vi "sonde data write to excel.vi"() -> ()   [LabVIEW 2016]
uses:
  Groundwater header.ctl
  activeXtest/activeXtest 2015 Folder/sample data row cluster.ctl
  activeXtest/activeXtest 2015 Folder/sonde cluster.ctl
  <vilib>/Utility/NIReport.llb/NI_report.lvclass
panel:
  out "Current Sample Sheet":string
  in  "stop":bool
  out "row max value":i32
  in  "Write Data Line":bool
  out "last occupied cell's name":string
  in  "Final Data for Sample Sheet?":bool
  in  "Sample Sheet Data Row Cluster":T1={"Head"=0.0, "Depth"=0.0, "comment string"="", "Sonde Data Cluster"={"Cumulative\nVolume"=100.0, "Specific\nConductance"=2.0, "Dissolved\nOxygen"=3.0, "pH"=4.0, "ORP"=5.0, "Temp"=26.0, "Salinity"=7.0}} {"Sonde Data Cluster"."Salinity" format="%_3g"; "Sonde Data Cluster"."Temp" format="%_2g"; "Sonde Data Cluster"."ORP" format="%_4g"; "Sonde Data Cluster"."pH" format="%_4g"; "Sonde Data Cluster"."Dissolved\nOxygen" format="%_4g"; "Sonde Data Cluster"."Specific\nConductance" format="%_4g"; "Sonde Data Cluster"."Cumulative\nVolume" format="%#_4g"}
  out "number of rows":i32
  in  "report file path 2":path=path "D:/Cascade/templates/Groundwater Profiling Log_empty_2.xlsx"
  out "data":string[][](array[string])
  out "Elapsed Time (ms)":u32
  in  "error in (no error)":errorcluster
  in  "Groundwater Header":T3
  out "Worksheet Names":string[](array[string])
  in  "template file path":path=path "D:/Cascade/templates/Groundwater Profiling Log_empty_labview_template.xlsx"
  out "error out":errorcluster
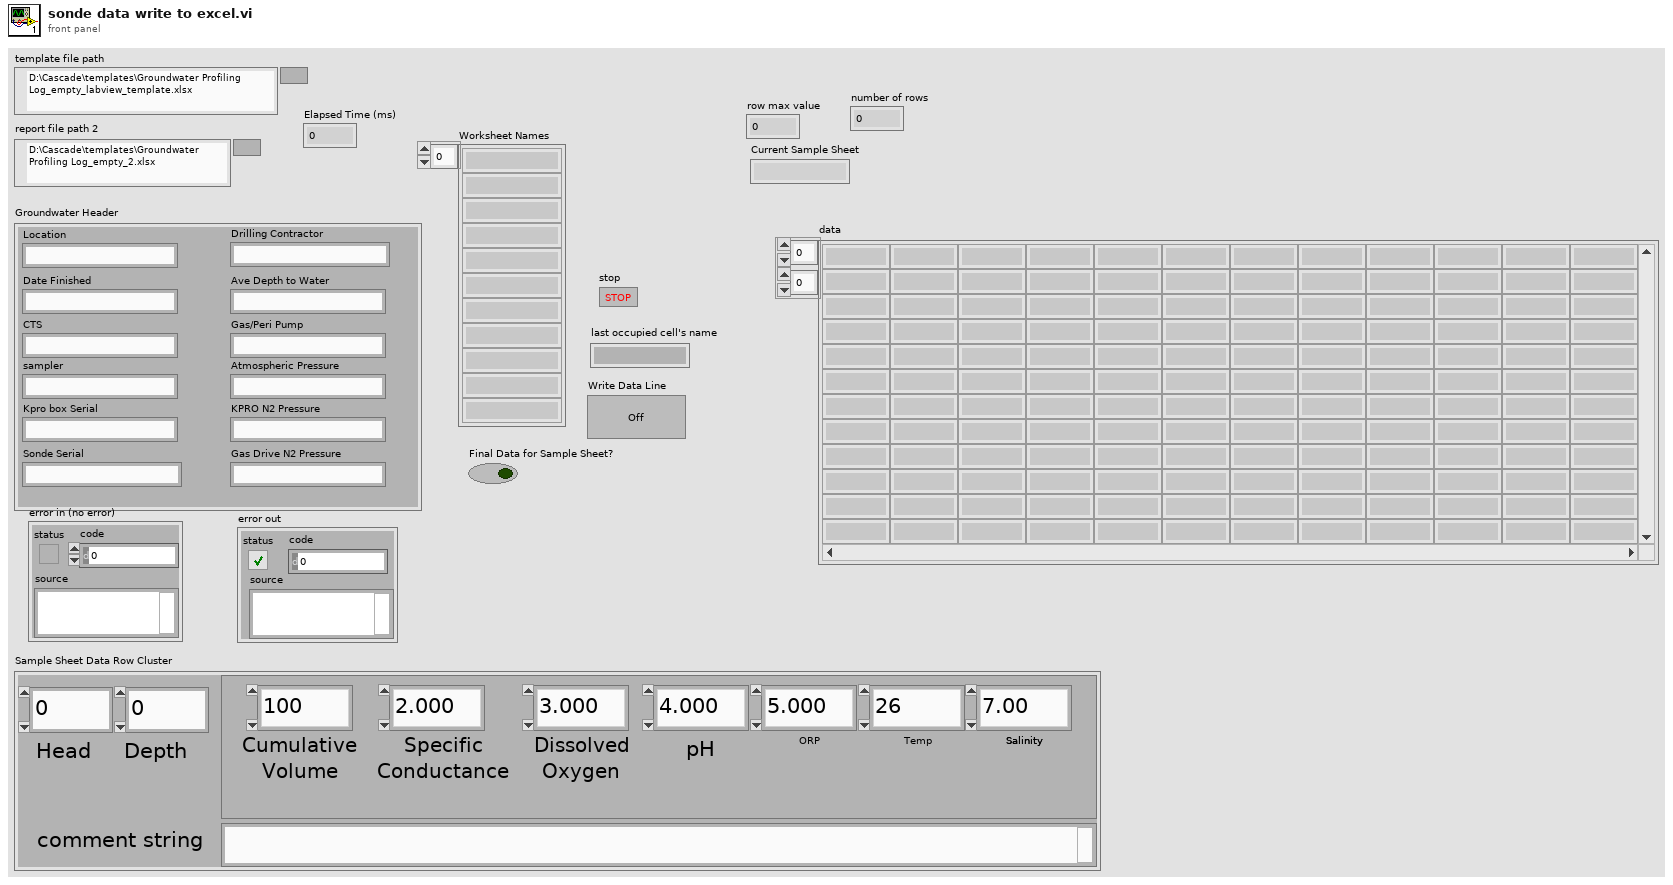
[diagram p1: front panel]
types:
  T1 = typedef "sample data row cluster.ctl" = cluster{"Head":dbl, "Depth":dbl, "comment string":string, "Sonde Data Cluster":T2}
  T2 = typedef "sonde cluster.ctl" = cluster{"Cumulative\nVolume":dbl, "Specific\nConductance":dbl, "Dissolved\nOxygen":dbl, "pH":dbl, "ORP":dbl, "Temp":dbl, "Salinity":dbl}
  T3 = typedef "Groundwater header.ctl" = cluster{"Location":string, "Date Finished":string, "CTS":string, "sampler":string, "Kpro box Serial ":string, "Sonde Serial":string, "Drilling Contractor":string, "Ave Depth to Water":string, "Gas/Peri Pump":string, "Atmospheric Pressure":string, "KPRO N2 Pressure":string, "Gas Drive N2 Pressure":string}
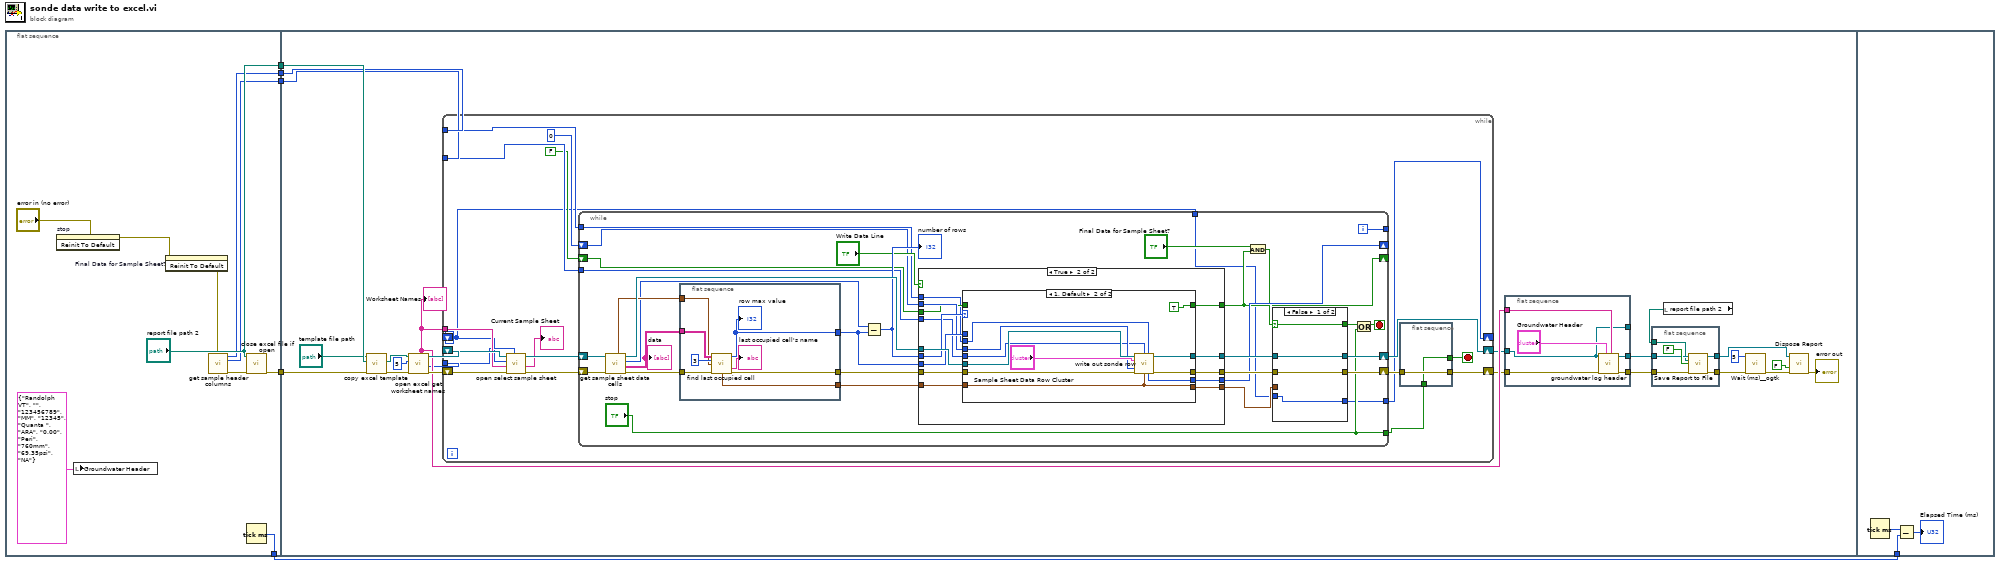
[diagram p0: block diagram]
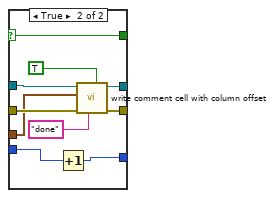
[diagram p4: hidden frame]
diagram:
  n1 = flat-sequence {
    tunnel: [w14] -> w5
    tunnel: [w12] -> w4
    tunnel: ["report file path 2"] -> w3
    tunnel: [w10] -> w2
    tunnel: [w9] -> w1
    tunnel: w4 -> [w26]
    tunnel: w3 -> [w24]
    tunnel: w2 -> [w19]
    tunnel: w1 -> [w18]
    tunnel: w5 -> [w161]
    frame #0 {
      n2 = invoke on="stop" class="Bool" method="Reinit To Default"(error in="error in (no error)") -> (error out=w6:errorcluster)  [unwired: 2 in, 2 out]
      n3 = local write "Groundwater Header"(T3 {"Location"="Randolph VT", "Date Finished"="", "CTS"="123456789", "sampler"="MM", "Kpro box Serial "="12345", "Sonde Serial"="Quanta ", "Drilling Contractor"="ARA", "Ave Depth to Water"="0.00", "Gas/Peri Pump"="Peri", "Atmospheric Pressure"="760mm", "KPRO N2 Pressure"="69.35psi", "Gas Drive N2 Pressure"="NA"} ("Groundwater Header 2")) -> ()
      n4 = invoke on="Final Data for Sample Sheet?" class="Bool" method="Reinit To Default"(error in=w6) -> (error out=w11:errorcluster)  [unwired: 2 in, 2 out]
      n5 = call "get sample header columns.vi"("error in (no error)"=w11) -> ("Column of Volume"=w10:i32, "Columns"=w9:i32[], "error out"=w8:errorcluster)  [unwired: 5 in, 7 out]
      n6 = call "close excel file if open.vi"("error in (no error)"=w8, "report file path in"="report file path 2") -> ("error out"=w12:errorcluster)  [unwired: 8 in, 1 out]
      n7 = Tick Count (ms)() -> (millisecond timer value=w14:u32)
    }
    frame #1 {
      n8 = call "copy excel template.vi"("error in (no error)"=w26, "report file path in"=w24, "template file path in"="template file path") -> ("error out"=w22:errorcluster, "report file path out"=w25:path)  [unwired: 7 in]
      n9 = call "open excel get worksheet names.vi"("error in (no error)"=w22, "milliseconds to wait"=u32 5, "report file path"=w25) -> ("error out"=w32:errorcluster, "Number of Sample Sheets"=w17:i32, "NI_report out"=w31:refnum<class "NI_report.lvclass">, "Worksheet Names"=w29:string[])  [unwired: 3 in, 2 out]
      "Worksheet Names" <- w29
      n10 = while {
        tunnel: w29 -> [w54]
        tunnel: w19 -> [w51]
        tunnel: w18 -> [w50]
        tunnel: w17 -> [w49]
        shift-right: [w45] -> w21
        shift-left: w32 -> [w56]
        shift-right: [w52] -> w20
        shift-left: w31 -> [w55]
        shift-right: [w41] -> _
        shift-left: 1 ("input 1") -> [w40]
        stop <- w48 stop-if-true
        n11 = call "open select sample sheet.vi"("Number of Sample Sheets"=w49, "error in (no error)"=w56, "Worksheet Names"=w54, "Active Sample Sheet"=w40, "NI_report in"=w55) -> ("error out"=w53:errorcluster, "Current Sample Sheet"=→"Current Sample Sheet":string, "NI_report out"=w57:refnum<class "NI_report.lvclass">)  [unwired: 4 in]
        n12 = while {
          shift-right: [w75] -> w52
          shift-left: w57 -> [w88]
          shift-right: [w77] -> w46
          shift-left: w53 -> [w79]
          tunnel: [w72] -> _
          shift-right: [w70] -> _
          shift-left: 0 ("row index") -> [w71]
          shift-right: [w64] -> _
          shift-left: FALSE ("x") -> [w67]
          tunnel: w51 -> [w66]
          tunnel: w50 -> [w65]
          tunnel: ["stop"] -> w44
          tunnel: w40 -> [w59]
          tunnel: [w58] -> w41
          i -> [w72]
          stop <- w61 stop-if-true
          n13 = call "get sample sheet data cells.vi"("error in (no error)"=w79, "NI_report in"=w88) -> ("error out"=w86:errorcluster, "data"=w80:string[][], "row"=w84:i32, "NI_report out"=w87:refnum<class "NI_report.lvclass">, "output cluster"=w85:cluster{"row":i32, "column":i32})  [unwired: 5 in]
          "data" <- w80
          n14 = flat-sequence {
            tunnel: w86 -> [w145]
            tunnel: w80 -> [w144]
            tunnel: w85 -> [w142]
            tunnel: [w141] -> w82
            tunnel: [w140] -> w81
            tunnel: [w139] -> w74
            frame #0 {
              n15 = call "find last occupied cell.vi"("data"=w144, "Header Rows to remove"=3, "sub array start"=w142, "error in (no error)"=w145) -> ("row max value"=w140:i32, "last occupied cell's name"=→"last occupied cell's name":string, "start of last occupied row"=w139:cluster{"row":i32, "column":i32}, "error out"=w141:errorcluster)  [unwired: 5 in, 3 out]
              "row max value" <- w140
            }
          }
          n16 = Subtract(x=w84, y=w81) -> (x-y=w83:i32)
          "number of rows" <- w83
          n17 = case shown="True" "Write Data Line" {
            tunnel: w87 -> [w93 w107]
            tunnel: w83 -> [_ w106]
            tunnel: w82 -> [w92 w105]
            tunnel: w81 -> [_ w104]
            tunnel: [w92 w103] -> w78
            tunnel: [w93 w102] -> w76
            tunnel: w74 -> [w90 w101]
            tunnel: w71 -> [w91 w100]
            tunnel: [w91 w99] -> w70
            tunnel: [w90 w98] -> w68
            tunnel: w67 -> [w89 w97]
            tunnel: [w89 w96] -> w64
            tunnel: w66 -> [_ w95]
            tunnel: w65 -> [_ w94]
            frame False {
            }
            frame True {
              n18 = case shown="1, Default" w106 {
                tunnel: [w111 w122] -> w103
                tunnel: [w112 w123] -> w102
                tunnel: w107 -> [w112 w121]
                tunnel: w101 -> [w109 w118]
                tunnel: w105 -> [w111 w115]
                tunnel: w104 -> [_ _]
                tunnel: w100 -> [w110 w119]
                tunnel: [w110 w116] -> w99
                tunnel: [w109 w118] -> w98
                tunnel: w97 -> [w108 _]
                tunnel: [w108 TRUE ("x")] -> w96
                tunnel: w95 -> [_ w114]
                tunnel: w94 -> [_ w113]
                frame 0 {
                }
                frame 1, Default {
                  n19 = call "write out sonde row.vi"("NI_report in"=w121, "Columns"=w113, "Column of Volume"=w114, "Sample Sheet Data Row Cluster"="Sample Sheet Data Row Cluster", "row index"=w119, "error in (no error)"=w115, "start of last occupied row"=w118) -> ("NI_report out"=w123:refnum<class "NI_report.lvclass">, "row index out"=w116:i32, "error out"=w122:errorcluster)  [unwired: 6 in]
                }
              }
            }
          }
          n20 = And(x="Final Data for Sample Sheet?", y=w64) -> (x .and. y?=w69:bool)
          n21 = case shown="False" w69 {
            selector: w69 -> [w125 w130]
            tunnel: w78 -> [w126 w137]
            tunnel: [w126 w136] -> w77
            tunnel: w76 -> [w127 w135]
            tunnel: [w127 w134] -> w75
            tunnel: w68 -> [_ w132]
            tunnel: [w125 w130] -> w62
            tunnel: w59 -> [w124 w129]
            tunnel: [w124 w128] -> w58
            frame False {
            }
            frame True {
              n22 = Increment(x=w129) -> (x+1=w128:i32)
              n23 = call "write comment cell with column offset.vi"("Column Relative?"=TRUE, "comment string"="done", "error in (no error)"=w137, "start of last occupied row"=w132, "NI_report in"=w135) -> ("error out"=w136:errorcluster, "NI_report out"=w134:refnum<class "NI_report.lvclass">)  [unwired: 5 in]
            }
          }
          n24 = Or(x=w62, y="stop") -> (x .or. y?=w61:bool)
        }
        n25 = flat-sequence {
          tunnel: [w146] -> w48
          tunnel: w46 -> [w147]
          tunnel: [w147] -> w45
          tunnel: w44 -> [w146]
          frame #0 {
          }
        }
      }
      n26 = flat-sequence {
        tunnel: w21 -> [w152]
        tunnel: [w151] -> w28
        tunnel: [w148] -> _
        tunnel: [w150] -> w30
        tunnel: w29 -> [w149]
        tunnel: w20 -> [w148]
        frame #0 {
          n27 = call "groundwater log header.vi"("Worksheet Names"=w149, "Groundwater Header"="Groundwater Header", "error in (no error)"=w152, "NI_report in"=w148) -> ("error out"=w151:errorcluster, "NI_report out"=w150:refnum<class "NI_report.lvclass">)  [unwired: 6 in]
        }
      }
      n28 = flat-sequence {
        tunnel: [w159] -> w39
        tunnel: [w158] -> w38
        tunnel: w28 -> [w156]
        tunnel: w30 -> [w155]
        tunnel: w27 -> [w154]
        frame #0 {
          n29 = call-dynamic "Save Report to File.vi"("report in"=w155, "report file path"=w154, "prompt to replace? (F)"=FALSE, "error in (no error)"=w156) -> ("report out"=w159:refnum<class "NI_report.lvclass">, "error out"=w158:errorcluster)  [unwired: 10 in]
        }
      }
      n30 = local read "report file path 2"() -> (w27:path)
      n31 = call <userlib>:"Wait (ms)__ogtk.vi"("error in (no error)"=w38, "milliseconds to wait"=u32 5) -> ("error out"=w35:errorcluster)  [unwired: 8 in, 1 out]
      n32 = call-dynamic "Dispose Report.vi"("report in"=w39, "save changes? (F)"=FALSE, "error in (no error)"=w35) -> ("error out"=→"error out":errorcluster)  [unwired: 12 in]
    }
    frame #2 {
      n33 = Tick Count (ms)() -> (millisecond timer value=w162:u32)
      n34 = Subtract(x=w162, y=w161) -> (x-y=→"Elapsed Time (ms)":u32)
    }
  }
